vi "AddProgram.vi"(0 "Program Interface in":refnum<class "Program Interface.lvclass">, 1 "addProgram":string, 5 "error in (no error)":errorcluster) -> (14 "Program Interface out":refnum<class "Program Interface.lvclass">, 19 "error out":errorcluster)   [LabVIEW 2016, in "Program Interface.lvclass"]
uses:
  Program Interface.lvclass
  C:/_Code/Development/UR LabVIEW Interface/Classes/Application Interface/Application Interface.lvclass
  Program Interface.lvclass/Program Interface.ctl
  Application/Application.lvclass
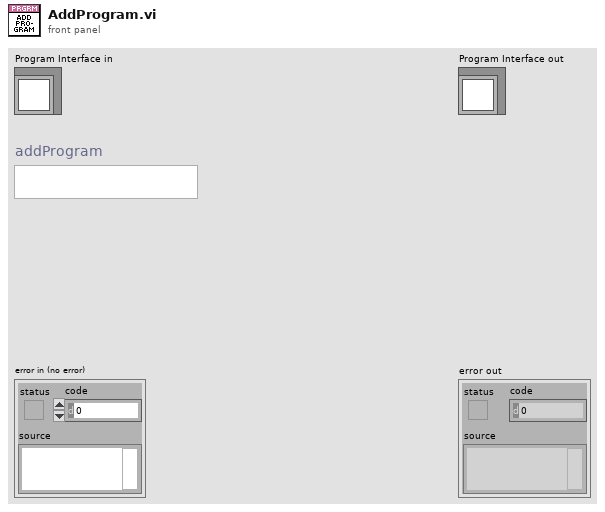
[diagram p1: front panel]
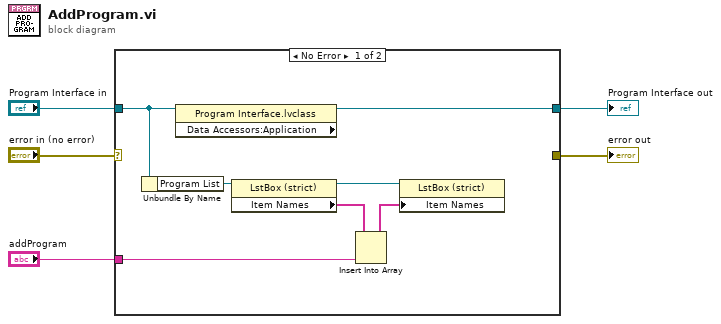
[diagram p0: block diagram]
diagram:
  n1 = case shown="No Error" "error in (no error)" {
    selector: "error in (no error)" -> [_ w14]
    tunnel: [_ w14] -> w4
    tunnel: [w12 w13] -> w2
    tunnel: "Program Interface in" -> [w11 w13]
    tunnel: "addProgram" -> [w6 _]
    frame No Error {
      n2 = Unbundle By Name(w11) -> ("Program List"=w10:refnum<vi>)
      n3 = property class="Program Interface.lvclass" props=["Data Accessors:Application"](reference=w11) -> (reference out=w12:refnum<class "Program Interface.lvclass">)  [unwired: 1 in, 2 out]
      n4 = property class="LstBox (strict)"(reference=w10) -> (reference out=w9:refnum<vi>, "Item Names"=w8:string[])  [unwired: 1 in, 1 out]
      n5 = Insert Into Array(array=w8, new element=w6) -> (w7:string[])  [unwired: 1 in]
      n6 = property class="LstBox (strict)"(reference=w9, "Item Names"=w7) -> ()  [unwired: 1 in, 2 out]
    }
    frame Error {
    }
  }
  "error out" <- w4
  "Program Interface out" <- w2
